vi "Lab Panel V6.00.vi"() -> ()   [LabVIEW 2017]
uses:
  SelectLAB0X-N.ctl
  SIG LAB0X-N.ctl
  Set LAB0X-N.ctl
  <vilib>/Platform/TimedLoop/XDataNode/timing_clust.ctl
  <vilib>/Platform/TimedLoop/XDataNode/nitl_modes.ctl
  <vilib>/Platform/TimedLoop/XDataNode/wakeup.ctl
  Global display 1.vi
  Global display 4.vi
  Global display 3.vi
  Global display 2.vi
  Global 1.vi
  <vilib>/platform/TimedLoop/XDataNode/XDataNode.xnode
  <vilib>/Platform/TimedLoop/XDataNode/XDNodeRunTimeDep.lvlib
panel:
  in  "path to JPEG file":path=path "C:/Users/Mike/Documents/Crabtree/Crabtree/Hardware/crabtree"
  out "Simulate IND":bool
  out "Amb Tp":dbl format="%#.0f"
  out "Tp Up":dbl
  out "network error":bool
  out "TEMP":bool
  out "AI":bool
  in  "stop all":bool
  in  "ADMIN":bool
  in  "Tab Control 2":T1(tab)
  out "SIG LAB05-2":T2 {"PF" format="%.2f"; "AMPS" format="%.1f"}
  out "SIG LAB05-1":T2 {"PF" format="%.2f"; "AMPS" format="%.1f"}
  out "SIG LAB04-2":T2 {"PF" format="%.2f"; "AMPS" format="%.1f"}
  out "SIG LAB04-1":T2 {"PF" format="%.2f"; "AMPS" format="%.1f"}
  out "SIG LAB03-2":T2 {"PF" format="%.2f"; "AMPS" format="%.1f"}
  out "SIG LAB03-1":T2 {"PF" format="%.2f"; "AMPS" format="%.1f"}
  out "SIG LAB02-2":T2 {"PF" format="%.2f"; "AMPS" format="%.1f"}
  in  "RUN LAB01-1":bool
  in  "O/I  LAB05-1":bool
  in  "O/I  LAB05-2":bool
  in  "O/I  LAB04-1":bool
  in  "O/I  LAB04-2":bool
  in  "O/I  LAB02-1":bool
  in  "O/I  LAB02-2":bool
  in  "O/I  LAB01-2":bool
  in  "O/I  LAB01-1":bool
  in  "O/I  LAB03-1":bool
  in  "RUN LAB05-2":bool
  in  "RUN LAB05-1":bool
  in  "RUN LAB04-2":bool
  in  "RUN LAB04-1":bool
  in  "RUN LAB03-2":bool
  in  "RUN LAB03-1":bool
  in  "RUN LAB02-2":bool
  in  "RUN LAB02-1":bool
  in  "RUN LAB01-2":bool
  in  "SELECT LAB05-2":T3
  in  "SELECT LAB05-1":T3
  in  "SELECT LAB04-2":T3
  in  "SELECT LAB04-1":T3
  in  "SELECT LAB03-2":T3
  in  "SELECT LAB03-1":T3
  in  "SELECT LAB02-2":T3
  in  "SELECT LAB02-1":T3
  in  "SELECT LAB01-2":T3
  in  "SELECT LAB01-1":T3
  in  "O/I  LAB03-2":bool
  out "SIG LAB01-1":T2 {"PF" format="%.2f"; "AMPS" format="%.1f"}
  out "SIG LAB01-2":T2 {"PF" format="%.2f"; "AMPS" format="%.1f"}
  out "SIG LAB02-1":T2 {"PF" format="%.2f"; "AMPS" format="%.1f"}
  out "DISP LAB05-2":T4 {"MINS" format="%.2g"}
  out "DISP LAB05-1":T4 {"MINS" format="%.2g"}
  out "DISP LAB04-2":T4 {"MINS" format="%.2g"}
  out "DISP LAB04-1":T4 {"MINS" format="%.2g"}
  out "DISP LAB03-2":T4 {"MINS" format="%.2g"}
  out "DISP LAB03-1":T4 {"MINS" format="%.2g"}
  in  "SET LAB05-2":T5={"NAME"="", "DESCRIPTION"="", "CYCLES"=5.0, "T-RISE mins"=0.0, "T-RISE deg C"=0.0} {"CYCLES" min=5.0 step=1.0}
  in  "SET LAB05-1":T5={"NAME"="", "DESCRIPTION"="", "CYCLES"=5.0, "T-RISE mins"=0.0, "T-RISE deg C"=0.0} {"CYCLES" min=5.0 step=1.0}
  in  "SET LAB04-2":T5={"NAME"="", "DESCRIPTION"="", "CYCLES"=5.0, "T-RISE mins"=0.0, "T-RISE deg C"=0.0} {"CYCLES" min=5.0 step=1.0}
  in  "SET LAB04-1":T5={"NAME"="", "DESCRIPTION"="", "CYCLES"=5.0, "T-RISE mins"=0.0, "T-RISE deg C"=0.0} {"CYCLES" min=5.0 step=1.0}
  in  "SET LAB03-2":T5={"NAME"="", "DESCRIPTION"="", "CYCLES"=5.0, "T-RISE mins"=0.0, "T-RISE deg C"=0.0} {"CYCLES" min=5.0 step=1.0}
  in  "SET LAB03-1":T5={"NAME"="", "DESCRIPTION"="", "CYCLES"=5.0, "T-RISE mins"=0.0, "T-RISE deg C"=0.0} {"CYCLES" min=5.0 step=1.0}
  out "DISP LAB02-2":T4 {"MINS" format="%.2g"}
  out "DISP LAB02-1":T4 {"MINS" format="%.2g"}
  in  "SET LAB02-2":T5={"NAME"="", "DESCRIPTION"="", "CYCLES"=5.0, "T-RISE mins"=0.0, "T-RISE deg C"=0.0} {"CYCLES" min=5.0 step=1.0}
  in  "SET LAB02-1":T5={"NAME"="", "DESCRIPTION"="", "CYCLES"=5.0, "T-RISE mins"=0.0, "T-RISE deg C"=0.0} {"CYCLES" min=5.0 step=1.0}
  out "RESULT LAB05-2":bool
  out "RESULT LAB05-1":bool
  out "RESULT LAB04-2":bool
  out "RESULT LAB04-1":bool
  out "RESULT LAB03-2":bool
  out "RESULT LAB03-1":bool
  out "RESULT LAB02-2":bool
  out "RESULT LAB02-1":bool
  out "RESULT LAB01-2":bool
  out "RESULT LAB01-1":bool
  in  "SET LAB01-1":T6={"NAME"="", "DESCRIPTION"="", "CYCLES"=5.0, "T-RISE mins"=0.0, "T-RISE deg C"=0.0} {"CYCLES" min=5.0 step=1.0}
  in  "SET LAB01-2":T5={"NAME"="", "DESCRIPTION"="", "CYCLES"=5.0, "T-RISE mins"=0.0, "T-RISE deg C"=0.0} {"CYCLES" min=5.0 step=1.0}
  out "DISP LAB01-1":T4 {"MINS" format="%.2g"}
  out "DISP LAB01-2":T4 {"MINS" format="%.2f"}
  out "TEMP RISE LAB05-2":cluster{"TL":dbl, "TN":dbl}
  out "TEMP RISE LAB05-1":cluster{"TL":dbl, "TN":dbl}
  out "TEMP RISE LAB04-2":cluster{"TL":dbl, "TN":dbl}
  out "TEMP RISE LAB04-1":cluster{"TL":dbl, "TN":dbl}
  out "TEMP RISE LAB03-2":cluster{"TL":dbl, "TN":dbl}
  out "TEMP RISE LAB03-1":cluster{"TL":dbl, "TN":dbl}
  out "TEMP RISE LAB02-2":cluster{"TL":dbl, "TN":dbl}
  out "TEMP RISE LAB02-1":cluster{"TL":dbl, "TN":dbl}
  out "TEMP RISE LAB01-2":cluster{"TL":dbl, "TN":dbl}
  out "TEMP RISE LAB01-1":cluster{"TL":dbl, "TN":dbl}
  out "JIG LAB05-2":bool
  out "JIG LAB05-1":bool
  out "JIG LAB04-2":bool
  out "JIG LAB04-1":bool
  out "JIG LAB03-2":bool
  out "JIG LAB03-1":bool
  out "JIG LAB02-2":bool
  out "JIG LAB02-1":bool
  out "JIG LAB01-2":bool
  out "JIG LAB01-1":bool
  out "TEMP START LAB01-1":cluster{"TL":dbl, "TN":dbl}
  out "TEMP START LAB02-1":cluster{"TL":dbl, "TN":dbl}
  out "TEMP START LAB03-1":cluster{"TL":dbl, "TN":dbl}
  out "TEMP START LAB04-1":cluster{"TL":dbl, "TN":dbl}
  out "TEMP START LAB01-2":cluster{"TL":dbl, "TN":dbl}
  out "TEMP START LAB02-2":cluster{"TL":dbl, "TN":dbl}
  out "TEMP START LAB03-2":cluster{"TL":dbl, "TN":dbl}
  out "TEMP START LAB04-2":cluster{"TL":dbl, "TN":dbl}
  out "TEMP START LAB05-2":cluster{"TL":dbl, "TN":dbl}
  out "TEMP START LAB05-1":cluster{"TL":dbl, "TN":dbl}
  out "LOG LAB05-2":string
  out "LOG LAB04-2":string
  out "LOG LAB03-2":string
  out "LOG LAB02-2":string
  out "LOG LAB01-2":string
  out "LOG LAB05-1":string
  out "LOG LAB04-1":string
  out "LOG LAB03-1":string
  out "LOG LAB02-1":string
  out "LOG LAB01-1":string
  in  "Tab charts":T7(tab)
  out "LAB01 VOLTS":dynamicdata(graph)
  out "LAB01 AMPS":dynamicdata(graph)
  out "LAB01 deg C":dynamicdata(graph)
  out "LAB02 VOLTS":dynamicdata(graph)
  out "LAB02 AMPS":dynamicdata(graph)
  out "LAB02 deg C":dynamicdata(graph)
  out "LAB03 VOLTS":dynamicdata(graph)
  out "LAB03 AMPS":dynamicdata(graph)
  out "LAB03 deg C":dynamicdata(graph)
  out "LAB04 VOLTS":dynamicdata(graph)
  out "LAB04 AMPS":dynamicdata(graph)
  out "LAB04 deg C":dynamicdata(graph)
  out "LAB05 VOLTS":dynamicdata(graph)
  out "LAB05 AMPS":dynamicdata(graph)
  out "LAB05 deg C":dynamicdata(graph)
  out "Reset Error":bool
  out "Er USB#2":dbl
  out "Er USB#1":dbl
  out "Er USB#0":dbl
  out "Resets Done":dbl
  out "Error USB #2":bool
  out "Error USB #1":bool
  out "Error USB #0":bool
  in  "MAIL SETTINGS":T8
  out "MAIL REPORT":string
  in  "TO (string):":string
  in  "Send Mail Now":bool
  in  "Auto Mail Send":bool
  in  "Network Directory":path
  in  "JIG ON TIME (S)":dbl=1.0 min=1.0 max=10.0 step=0.5 format="%.1g"
  in  "JIG OFF TIME (S)":dbl=2.0 min=2.0 max=10.0 step=0.5 format="%.1g"
  in  "Reset Measuring":bool
  out "path":path
  out "JIG RELAY CYCLES":T9
  out "ON L05-2":cluster{"amps":dbl, "volts":dbl, "pf":dbl}
  out "ON L05-1":cluster{"amps":dbl, "volts":dbl, "pf":dbl}
  out "FAIL LAB05-2":cluster{"LO":dbl, "HI":dbl}
  out "FAIL LAB05-1":cluster{"LO":dbl, "HI":dbl}
  out "FAIL LAB04-2":cluster{"LO":dbl, "HI":dbl}
  out "FAIL LAB04-1":cluster{"LO":dbl, "HI":dbl}
  out "FAIL LAB03-2":cluster{"LO":dbl, "HI":dbl}
  out "FAIL LAB03-1":cluster{"LO":dbl, "HI":dbl}
  out "FAIL LAB02-2":cluster{"LO":dbl, "HI":dbl}
  out "FAIL LAB02-1":cluster{"LO":dbl, "HI":dbl}
  out "FAIL LAB01-2":cluster{"LO":dbl, "HI":dbl}
  out "FAIL LAB01-1":cluster{"LO":dbl, "HI":dbl}
  out "ON L01-1":cluster{"amps":dbl, "volts":dbl, "pf":dbl}
  out "ON L01-2":cluster{"amps":dbl, "volts":dbl, "pf":dbl}
  out "ON L02-1":cluster{"amps":dbl, "volts":dbl, "pf":dbl}
  out "ON L02-2":cluster{"amps":dbl, "volts":dbl, "pf":dbl}
  out "ON L03-1":cluster{"amps":dbl, "volts":dbl, "pf":dbl}
  out "ON L03-2":cluster{"amps":dbl, "volts":dbl, "pf":dbl}
  out "ON L04-1":cluster{"amps":dbl, "volts":dbl, "pf":dbl}
  out "ON L04-2":cluster{"amps":dbl, "volts":dbl, "pf":dbl}
  in  "Open Com Port":bool
  out "LA05-2 (TN)":bool
  out "LA05-2 (TL)":bool
  out "LA05-1 (TN)":bool
  out "LA05-1 (TL)":bool
  out "LA04-2 (TN)":bool
  out "LA04-2 (TL)":bool
  out "LA04-1 (TN)":bool
  out "LA04-1 (TL)":bool
  out "LA03-2 (TN)":bool
  out "LA03-2 (TL)":bool
  out "LA03-1 (TN)":bool
  out "LA03-1 (TL)":bool
  out "LA02-2 (TN)":bool
  out "LA02-2 (TL)":bool
  out "LA02-1 (TN)":bool
  out "LA02-1 (TL)":bool
  out "LA01-2 (TN)":bool
  out "LA01-2 (TL)":bool
  out "LA01-1 (TN)":bool
  out "LA01-1 (TL)":bool
  out "TEMP LA05":T10
  out "TEMP LA04":T10
  out "TEMP LA03":T10
  out "TEMP LA02":T10
  out "TEMP LA01":T10
  out "Ref deg C":dbl format="%#.0f"
  out "Temp read loop":dbl
  out "Com Port Status":bool
  out "Com setup loops":i32
  out "VISA Com out":refnum<visa-resource-name>
  in  "Select COM port":refnum<visa-resource-name>="COM6"
  in  "Read Temp":bool
  out "Error Temp":bool
  out "AI Task":bool
  out "AI Task2":dbl
  out "AI Task1":dbl
  out "AI Task0":dbl
  out "Total USB resets":dbl
  in  "Auto Reset":bool
  in  "Mail Test File To:":string
  in  "Mail Test Fail":bool
  out "graph flag":bool
  in  "Temp Test Cal":dbl
  in  "Amps Fail level":dbl
  in  "Fail Loops":dbl
  out "Save JC":bool
  in  "Simulate":bool
  in  "Temp Value":dbl
  in  "Temp Delay Lps":dbl
  in  "SAMPLES":dbl
  in  "RATE (Hz)":dbl
  in  "JIG TEST":T11
  in  "C drive data root dir":path
  out "run lab05-2":bool
  out "run lab05-1":bool
  out "run lab04-2":bool
  out "run lab04-1":bool
  out "run lab03-2":bool
  out "run lab03-1":bool
  out "run lab02-2":bool
  out "run lab02-1":bool
  out "run lab01-2":bool
  out "run lab01-1":bool
  in  "Tab Control":T12(tab)
  out "LAB01-2 (GRAPH)":dynamicdata(graph)
  out "LAB01-1 (GRAPH)":dynamicdata(graph)
  out "LAB02-2 (GRAPH)":dynamicdata(graph)
  out "LAB02-1 (GRAPH)":dynamicdata(graph)
  out "LAB03-2 (GRAPH)":dynamicdata(graph)
  out "LAB03-1 (GRAPH)":dynamicdata(graph)
  out "LAB04-2 (GRAPH)":dynamicdata(graph)
  out "LAB04-1 (GRAPH)":dynamicdata(graph)
  out "LAB05-2 (GRAPH)":dynamicdata(graph)
  out "LAB05-1 (GRAPH)":dynamicdata(graph)
  out "Any Test Running":bool
  out "Read Time":dbl
  out "LAB05 TEMP":T13
  out "LAB04 TEMP":T13
  out "LAB02 TEMP":T13
  out "LAB01 TEMP":T13
  out "LAB03 TEMP":T13
  out "LAB05-TP":bool
  out "LAB04-TP":bool
  out "LAB03-TP":bool
  out "LAB02-TP":bool
  out "LAB01-TP":bool
  out "Analog error":bool
  out "USB OUT 0":bool[](array[boolean])
  out "USB OUT 1":bool[](array[boolean])
  out "USB OUT 2":bool[](array[boolean])
  in  "Ambient Volts":dbl format="%.2f"
  in  "PF":dbl min=0.0 max=1.0 step=0.1 format="%#.1f"
  in  "VOLTS":dbl
  in  "OFF amps":dbl min=0.0 max=100.0 step=0.1 format="%#.1f"
  in  "ON amps":dbl
  in  "LAB deg C":T14
  out "AI data 0":waveform(dbl)[](array[waveform])
  out "AI data 1":waveform(dbl)[](array[waveform])
  out "AI data 2":waveform(dbl)[](array[waveform])
  out "AI Error":errorcluster[](array[cluster])
  out "AI loop time":dbl format="%.6g"
  out "loops":dbl
  out "on loops":dbl format="%#.0f"
  out "off loops":dbl format="%#.0f"
  out "jig cycle":dbl
  out "TDMS LAB01-1":refnum<k34>
  out "data file error":errorcluster
  out "TDMS LAB02-1":refnum<k34>
  out "TDMS LAB01-2":refnum<k34>
  out "TDMS LAB02-2":refnum<k34>
  out "TDMS LAB03-1":refnum<k34>
  out "TDMS LAB03-2":refnum<k34>
  out "TDMS LAB04-1":refnum<k34>
  out "TDMS LAB04-2":refnum<k34>
  out "TDMS LAB05-1":refnum<k34>
  out "TDMS LAB05-2":refnum<k34>
  out "mail control":string
  out "File Time Stamp":timestamp
  in  "stop":bool
  out "deg C (volts)":dbl
  out "Application Directory":path
  out "TEMP REF cal":dbl
  out "CAL LAB01":T15 {"2 (TN) cal" min=0.0 step=0.01 format="%.2f"; "2 (TL) cal" min=0.0 step=0.01 format="%.2f"; "2 (PF) cal" min=0.0 step=0.01 format="%.2f"; "2 (V) cal" min=0.0 step=0.01 format="%.2f"; "2 (A) cal" min=0.0 step=0.01 format="%.2f"; "1 (TN) cal" min=0.0 step=0.01 format="%.2f"; "1 (TL) cal" min=0.0 step=0.01 format="%.2f"; "1 (PF) cal" min=0.0 step=0.01 format="%.2f"; "1 (V) cal" min=0.0 step=0.01 format="%.2f"; "1  (A) cal" min=0.0 step=0.01 format="%.2f"}
  out "CAL LAB03":T15 {"2 (TN) cal" min=0.0 step=0.01 format="%.2f"; "2 (TL) cal" min=0.0 step=0.01 format="%.2f"; "2 (PF) cal" min=0.0 step=0.01 format="%.2f"; "2 (V) cal" min=0.0 step=0.01 format="%.2f"; "2 (A) cal" min=0.0 step=0.01 format="%.2f"; "1 (TN) cal" min=0.0 step=0.01 format="%.2f"; "1 (TL) cal" min=0.0 step=0.01 format="%.2f"; "1 (PF) cal" min=0.0 step=0.01 format="%.2f"; "1 (V) cal" min=0.0 step=0.01 format="%.2f"; "1  (A) cal" min=0.0 step=0.01 format="%.2f"}
  out "CAL LAB02":T16 {"2 (TN) cal" min=0.0 step=0.01 format="%.2f"; "2 (TL) cal" min=0.0 step=0.01 format="%.2f"; "2 (PF) cal" min=0.0 step=0.01 format="%.2f"; "2 (V) cal" min=0.0 step=0.01 format="%.2f"; "2 (A) cal" min=0.0 step=0.01 format="%.2f"; "1 (TN) cal" min=0.0 step=0.01 format="%.2f"; "1 (TL) cal" min=0.0 step=0.01 format="%.2f"; "1 (PF) cal" min=0.0 step=0.01 format="%.2f"; "1 (V) cal" min=0.0 step=0.01 format="%.2f"; "1 (A) cal" min=0.0 step=0.01 format="%.2f"}
  out "CAL LAB05":T15 {"2 (TN) cal" min=0.0 step=0.01 format="%.2f"; "2 (TL) cal" min=0.0 step=0.01 format="%.2f"; "2 (PF) cal" min=0.0 step=0.01 format="%.2f"; "2 (V) cal" min=0.0 step=0.01 format="%.2f"; "2 (A) cal" min=0.0 step=0.01 format="%.2f"; "1 (TN) cal" min=0.0 step=0.01 format="%.2f"; "1 (TL) cal" min=0.0 step=0.01 format="%.2f"; "1 (PF) cal" min=0.0 step=0.01 format="%.2f"; "1 (V) cal" min=0.0 step=0.01 format="%.2f"; "1  (A) cal" min=0.0 step=0.01 format="%.2f"}
  out "CAL LAB04":T15 {"2 (TN) cal" min=0.0 step=0.01 format="%.2f"; "2 (TL) cal" min=0.0 step=0.01 format="%.2f"; "2 (PF) cal" min=0.0 step=0.01 format="%.2f"; "2 (V) cal" min=0.0 step=0.01 format="%.2f"; "2 (A) cal" min=0.0 step=0.01 format="%.2f"; "1 (TN) cal" min=0.0 step=0.01 format="%.2f"; "1 (TL) cal" min=0.0 step=0.01 format="%.2f"; "1 (PF) cal" min=0.0 step=0.01 format="%.2f"; "1 (V) cal" min=0.0 step=0.01 format="%.2f"; "1  (A) cal" min=0.0 step=0.01 format="%.2f"}
  out "cal file error out":errorcluster
  in  "SET (cal)":bool
  out "AI Data 0":waveform(dbl)[](graph)
  out "AI Data 1":waveform(dbl)[](graph)
  out "AI Data 2":waveform(dbl)[](graph)
  # "http://Mike:8000/Lab%20Panel%20V6.0.html"
  # "LAB01"
  # "LAB02"
  # "LAB03"
  # "LAB04"
  # "LAB05"
  # "LAB01"
  # "LAB02"
  # "LAB03"
  # "LAB04"
  # "LAB05"
  # "PANEL ID / DATE / TIME / NAME / DESCRIPTION / CYCLES / TEST TIME / STATUS"
  # "PANEL ID / DATE / TIME / NAME / DESCRIPTION / CYCLES / TEST TIME / STATUS"
  # "http://This IP:8000/Lab_Panel"
  # "(Enter recipients address seperated by comma)"
  # "JIG SET"
  # "Temperature circuits \ndetected at start up."
  # "PANEL CONTROL TO BE ON"
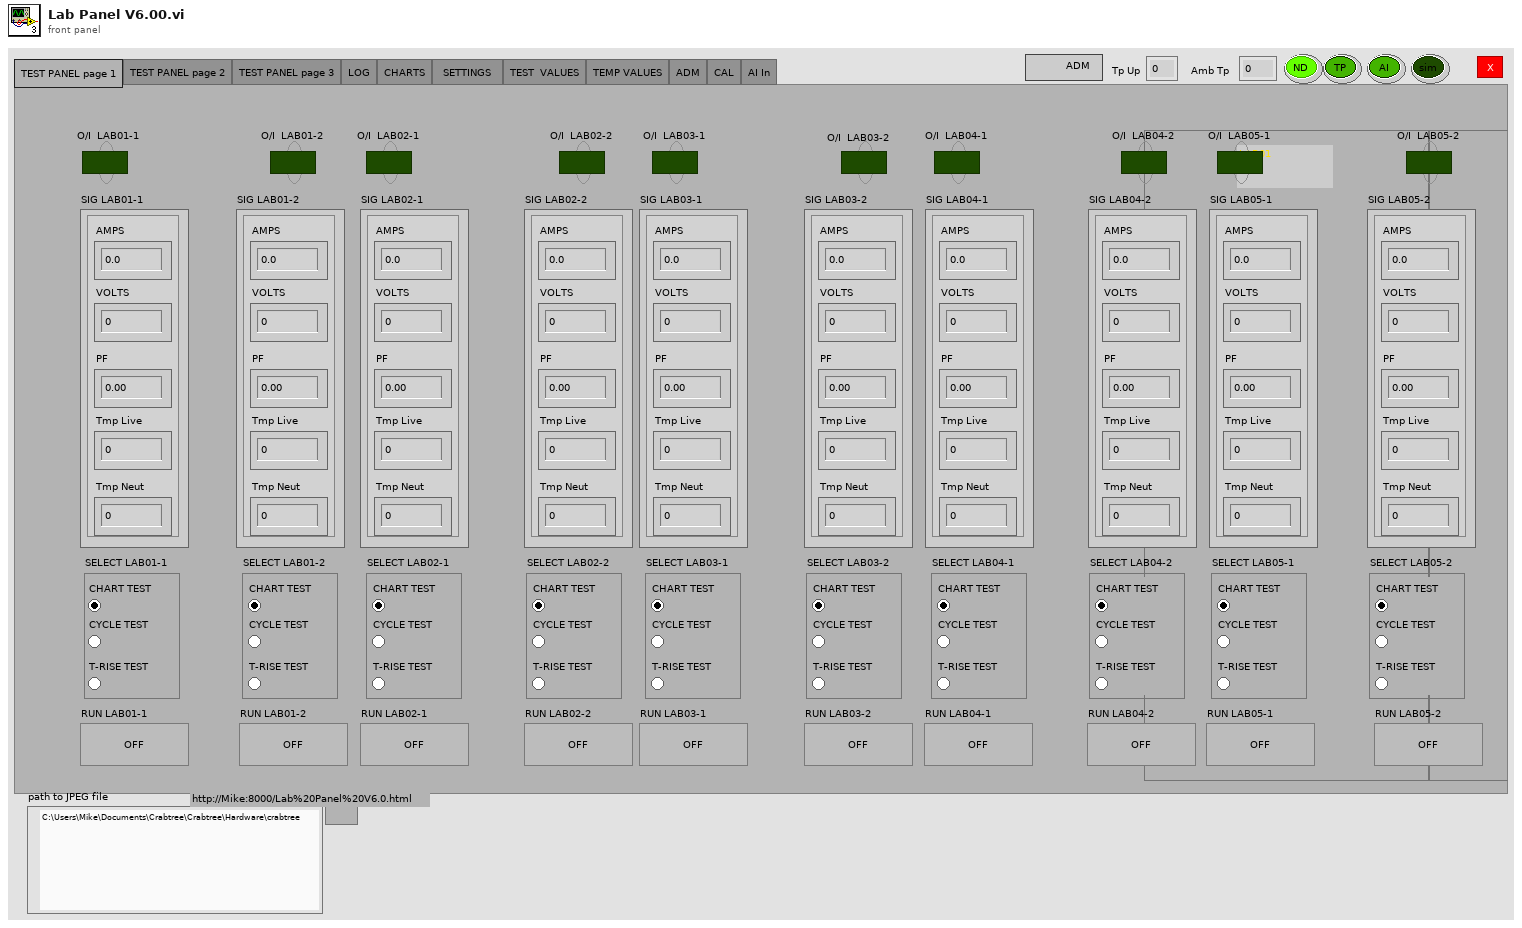
[diagram p1: front panel]
types:
  T1 = enum32{"TEST PANEL page 1", "TEST PANEL page 2", "TEST PANEL page 3", "LOG", "CHARTS", "SETTINGS   ", "TEST  VALUES", "TEMP VALUES", "ADM", "CAL", "AI In"}
  T2 = typedef "SIG LAB0X-N.ctl" = cluster{"AMPS":dbl, "VOLTS":dbl, "PF":dbl, "Tmp Live":dbl, "Tmp Neut":dbl}
  T3 = typedef "SelectLAB0X-N.ctl" = enum32{"CHART TEST", "CYCLE TEST", "T-RISE TEST"}
  T4 = cluster{"CYCLE":dbl, "MINS":dbl, "STATUS":string}
  T5 = cluster{"NAME":string, "DESCRIPTION":string, "CYCLES":dbl, "T-RISE mins":dbl, "T-RISE deg C":dbl}
  T6 = typedef "Set LAB0X-N.ctl" = cluster{"NAME":string, "DESCRIPTION":string, "CYCLES":dbl, "T-RISE mins":dbl, "T-RISE deg C":dbl}
  T7 = enum32{"LAB01", "LAB02", "LAB03", "LAB04", "LAB05"}
  T8 = cluster{"OUT SERVER ADDRESS":string, "FROM ACCOUNT":string, "USER NAME":string, "PASSWORD":string, "TEST MAIL":bool, "TEST MAIL STATUS":string, "mail error":errorcluster}
  T9 = cluster{"LAB01-1":dbl, "LAB01-2":dbl, "LAB02-1":dbl, "LAB02-2":dbl, "LAB03-1":dbl, "LAB03-2":dbl, "LAB04-1":dbl, "LAB04-2":dbl, "LAB05-1":dbl, "LAB05-2":dbl}
  T10 = cluster{"TL-1":dbl, "TN-1":dbl, "TL-2":dbl, "TN-2":dbl, "TL -1COUNT":dbl, "TN-1 COUNT":dbl, "TL-2 COUNT":dbl, "TN-2 COUNT":dbl}
  T11 = cluster{" LAB01-1":bool, " LAB01-2":bool, "LAB02-1":bool, " LAB02-2":bool, "LAB03-1":bool, "LAB03-2":bool, "LAB04-1":bool, "LAB04-2":bool, "LAB05-1":bool, "LAB05-2":bool}
  T12 = enum32{"LAB01", "LAB02", "LAB03", "LAB04", "LAB05", "TEMPERATURE", "GENERAL INFO", "Simulate", "AI Data Out"}
  T13 = cluster{"T1 Live":dbl, "T1 Neut":dbl, "T2 Live":dbl, "T2 Neut":dbl, "ID":dbl, "ER":dbl}
  T14 = cluster{"1 TL":dbl, "1 TN":dbl, "2 TL":dbl, "2 TN":dbl, "ID":dbl, "ER":dbl}
  T15 = cluster{"1  (A) cal":dbl, "1 (V) cal":dbl, "1 (PF) cal":dbl, "1 (TL) cal":dbl, "1 (TN) cal":dbl, "2 (A) cal":dbl, "2 (V) cal":dbl, "2 (PF) cal":dbl, "2 (TL) cal":dbl, "2 (TN) cal":dbl}
  T16 = cluster{"1 (A) cal":dbl, "1 (V) cal":dbl, "1 (PF) cal":dbl, "1 (TL) cal":dbl, "1 (TN) cal":dbl, "2 (A) cal":dbl, "2 (V) cal":dbl, "2 (PF) cal":dbl, "2 (TL) cal":dbl, "2 (TN) cal":dbl}
  T17 = enum8{"Enabled", "Disabled", "Disabled and Grayed Out"}
  T18 = enum16{"open", "replace", "create", "open or create", "replace or create", "replace or create with confirmation"}
  T19 = typedef "XDNodeRunTimeDep.lvlib/timing_clust.ctl" = cluster{"Expected End [f-1]":u64, "Actual End [f-1]":u64, "Finished Late? [f-1]":bool, "Expected End [i-1]":u64, "Actual End [i-1]":u64, "Finished Late? [i-1]":bool, "Expected Start [i]":u64, "Actual Start [i]":u64, "Expected Start [f]":u64, "Actual Start [f]":u64, "Source Name":string, "Structure Name":string, "Period":i64, "Deadline":i64, "Offset":i64, "Start":i64, "Priority":i32, "Timeout":i32, "Mode":T20, "Wakeup Reason":T21, "Error":errorcluster, "Source Type":string, "Secondary Source Type":string, "Global End Time":u64, "Global Start Time":u64, "Frame Duration":u64, "Iteration Duration":u64, "Assigned CPU":i32, "I/O Scan Engine Mode":u32}
  T20 = typedef "XDNodeRunTimeDep.lvlib/nitl_modes.ctl" = enum32{"No Change", "Process missed periods, maintain original phase", "Discard missed periods, maintain original phase", "Process missed periods, ignore original phase", "Discard missed periods, ignore original phase"}
  T21 = typedef "XDNodeRunTimeDep.lvlib/wakeup.ctl" = enum32{"Normal", "Aborted", "Asynchronous wakeup", "Timing source error", "Timed loop error", "Timeout"}
  T22 = enum16{"open", "open or create", "create or replace", "create", "open (read-only)"}
  T23 = cluster{"status":string, "mail server":string, "mail from":string, "mail to":string, "mail file":bool}
  T24 = cluster{"SET LAB01-1":T6, "SET LAB01-2":cluster{"NAME":string, "DESCRIPTION":string, "CYCLES":dbl, "T-RISE mins":dbl, "T-RISE deg C":dbl}, "SET LAB02-1":cluster{"NAME":string, "DESCRIPTION":string, "CYCLES":dbl, "T-RISE mins":dbl, "T-RISE deg C":dbl}, "SET LAB02-2":cluster{"NAME":string, "DESCRIPTION":string, "CYCLES":dbl, "T-RISE mins":dbl, "T-RISE deg C":dbl}, "SET LAB03-1":cluster{"NAME":string, "DESCRIPTION":string, "CYCLES":dbl, "T-RISE mins":dbl, "T-RISE deg C":dbl}, "SET LAB03-2":cluster{"NAME":string, "DESCRIPTION":string, "CYCLES":dbl, "T-RISE mins":dbl, "T-RISE deg C":dbl}, "SET LAB04-1":cluster{"NAME":string, "DESCRIPTION":string, "CYCLES":dbl, "T-RISE mins":dbl, "T-RISE deg C":dbl}, "SET LAB04-2":cluster{"NAME":string, "DESCRIPTION":string, "CYCLES":dbl, "T-RISE mins":dbl, "T-RISE deg C":dbl}, "SET LAB05-1":cluster{"NAME":string, "DESCRIPTION":string, "CYCLES":dbl, "T-RISE mins":dbl, "T-RISE deg C":dbl}, "SET LAB05-2":cluster{"NAME":string, "DESCRIPTION":string, "CYCLES":dbl, "T-RISE mins":dbl, "T-RISE deg C":dbl}, "Network Directory":path, "C drive data root dir":path, "RATE (Hz)":dbl, "SAMPLES":dbl, "Select COM port":refnum<visa-resource-name>, "Temp Delay Lps":dbl, "Temp Value":dbl, "Fail Loops":dbl, "Temp Test Cal":dbl, "Amps Fail level":dbl, "Mail Test File To:":string, "Mail Test Fail":bool}
  T25 = cluster{"MAIL SETTINGS":cluster{"OUT SERVER ADDRESS":string, "FROM ACCOUNT":string, "USER NAME":string, "PASSWORD":string, "TEST MAIL":bool, "TEST MAIL STATUS":string, "mail error":errorcluster}, "Auto Mail Send":bool, string}
  T26 = cluster{"id1":bool, "id2":bool, "id3":bool, "id4":bool, "id5":bool}
  T27 = cluster{"T1":dbl, "T2":dbl, "T3":dbl, "T4":dbl, "ID":dbl, "ER":dbl}
  T28 = typedef "imagedata.ctl" = cluster{"image type":i32, "image depth":i32, "image":u8[], "mask":u8[], "colors":u32[], "Rectangle":cluster{"left":i16, "top":i16, "right":i16, "bottom":i16}}
  T29 = cluster{"STATUS":string, "OUT SERVER ADDRESS":string, "FROM ACCOUNT":string, "Mail Test File To:":string, "Mail Test Fail":bool}
  T30 = cluster{"LAB01-1 (A)":dbl, "LAB01-1 (V)":dbl, "LAB01-1 (PF)":dbl, "LAB01-2 (A)":dbl, "LAB01-2 (V)":dbl, "LAB01-2 (PF)":dbl}
  T31 = cluster{"LAB02-1 (A)":dbl, "LAB02-1 (V)":dbl, "LAB02-1 (PF)":dbl, "LAB02-2 (A)":dbl, "LAB02-2 (V)":dbl, "LAB02-2 (PF)":dbl}
  T32 = cluster{"LAB03-1 (A)":dbl, "LAB03-1 (V)":dbl, "LAB03-1 (PF)":dbl, "LAB03-2 (A)":dbl, "LAB03-2 (V)":dbl, "LAB03-2 (PF)":dbl}
  T33 = cluster{"LAB04-1 (A)":dbl, "LAB04-1 (V)":dbl, "LAB04-1 (PF)":dbl, "LAB04-2 (A)":dbl, "LAB04-2 (V)":dbl, "LAB04-2 (PF)":dbl}
  T34 = cluster{"LAB05-1 (A)":dbl, "LAB05-1 (V)":dbl, "LAB05-1 (PF)":dbl, "LAB05-2 (A)":dbl, "LAB05-2 (V)":dbl, "LAB05-2 (PF)":dbl}
  T35 = cluster{"OFF amps":dbl, "VOLTS":dbl, "PF":dbl, "OFF amps":dbl, "VOLTS":dbl, "PF":dbl}
  T36 = cluster{"FAIL LAB01-1":cluster{"LO":dbl, "HI":dbl}, "SIG LAB01-1":T2, "TEMP START LAB01-1":cluster{"TL":dbl, "TN":dbl}, "DISP LAB01-1":cluster{"CYCLE":dbl, "MINS":dbl, "STATUS":string}, "SET LAB01-1":T6, "TDMS LAB01-1":refnum<k34>}
  T37 = cluster{"FAIL LAB01-2":cluster{"LO":dbl, "HI":dbl}, "SIG LAB01-2":T2, "TEMP START LAB01-2":cluster{"TL":dbl, "TN":dbl}, "DISP LAB01-2":cluster{"CYCLE":dbl, "MINS":dbl, "STATUS":string}, "SET LAB01-2":cluster{"NAME":string, "DESCRIPTION":string, "CYCLES":dbl, "T-RISE mins":dbl, "T-RISE deg C":dbl}, "TDMS LAB01-2":refnum<k34>}
  T38 = cluster{"FAIL LAB02-1":cluster{"LO":dbl, "HI":dbl}, "SIG LAB02-1":T2, "TEMP START LAB02-1":cluster{"TL":dbl, "TN":dbl}, "DISP LAB02-1":cluster{"CYCLE":dbl, "MINS":dbl, "STATUS":string}, "SET LAB02-1":cluster{"NAME":string, "DESCRIPTION":string, "CYCLES":dbl, "T-RISE mins":dbl, "T-RISE deg C":dbl}, "TDMS LAB02-1":refnum<k34>}
  T39 = cluster{"FAIL LAB02-2":cluster{"LO":dbl, "HI":dbl}, "SIG LAB02-2":T2, "TEMP START LAB02-2":cluster{"TL":dbl, "TN":dbl}, "DISP LAB02-2":cluster{"CYCLE":dbl, "MINS":dbl, "STATUS":string}, "SET LAB02-2":cluster{"NAME":string, "DESCRIPTION":string, "CYCLES":dbl, "T-RISE mins":dbl, "T-RISE deg C":dbl}, "TDMS LAB02-2":refnum<k34>}
  T40 = cluster{"FAIL LAB03-1":cluster{"LO":dbl, "HI":dbl}, "SIG LAB03-1":T2, "TEMP START LAB03-1":cluster{"TL":dbl, "TN":dbl}, "DISP LAB03-1":cluster{"CYCLE":dbl, "MINS":dbl, "STATUS":string}, "SET LAB03-1":cluster{"NAME":string, "DESCRIPTION":string, "CYCLES":dbl, "T-RISE mins":dbl, "T-RISE deg C":dbl}, "TDMS LAB03-1":refnum<k34>}
  T41 = cluster{"FAIL LAB03-2":cluster{"LO":dbl, "HI":dbl}, "SIG LAB03-2":T2, "TEMP START LAB03-2":cluster{"TL":dbl, "TN":dbl}, "DISP LAB03-2":cluster{"CYCLE":dbl, "MINS":dbl, "STATUS":string}, "SET LAB03-2":cluster{"NAME":string, "DESCRIPTION":string, "CYCLES":dbl, "T-RISE mins":dbl, "T-RISE deg C":dbl}, "TDMS LAB03-2":refnum<k34>}
  T42 = cluster{"FAIL LAB04-1":cluster{"LO":dbl, "HI":dbl}, "SIG LAB04-1":T2, "TEMP START LAB04-1":cluster{"TL":dbl, "TN":dbl}, "DISP LAB04-1":cluster{"CYCLE":dbl, "MINS":dbl, "STATUS":string}, "SET LAB04-1":cluster{"NAME":string, "DESCRIPTION":string, "CYCLES":dbl, "T-RISE mins":dbl, "T-RISE deg C":dbl}, "TDMS LAB04-1":refnum<k34>}
  T43 = cluster{"FAIL LAB04-2":cluster{"LO":dbl, "HI":dbl}, "SIG LAB04-2":T2, "TEMP START LAB04-2":cluster{"TL":dbl, "TN":dbl}, "DISP LAB04-2":cluster{"CYCLE":dbl, "MINS":dbl, "STATUS":string}, "SET LAB04-2":cluster{"NAME":string, "DESCRIPTION":string, "CYCLES":dbl, "T-RISE mins":dbl, "T-RISE deg C":dbl}, "TDMS LAB04-2":refnum<k34>}
  T44 = cluster{"FAIL LAB05-1":cluster{"LO":dbl, "HI":dbl}, "SIG LAB05-1":T2, "TEMP START LAB05-1":cluster{"TL":dbl, "TN":dbl}, "DISP LAB05-1":cluster{"CYCLE":dbl, "MINS":dbl, "STATUS":string}, "SET LAB05-1":cluster{"NAME":string, "DESCRIPTION":string, "CYCLES":dbl, "T-RISE mins":dbl, "T-RISE deg C":dbl}, "TDMS LAB05-1":refnum<k34>}
  T45 = cluster{"FAIL LAB05-2":cluster{"LO":dbl, "HI":dbl}, "SIG LAB05-2":T2, "TEMP START LAB05-2":cluster{"TL":dbl, "TN":dbl}, "DISP LAB05-2":cluster{"CYCLE":dbl, "MINS":dbl, "STATUS":string}, "SET LAB05-2":cluster{"NAME":string, "DESCRIPTION":string, "CYCLES":dbl, "T-RISE mins":dbl, "T-RISE deg C":dbl}, "TDMS LAB05-2":refnum<k34>}
  T46 = cluster{"MAIL SETTINGS":cluster{"OUT SERVER ADDRESS":string, "FROM ACCOUNT":string, "USER NAME":string, "PASSWORD":string, "TEST MAIL":bool, "TEST MAIL STATUS":string, "mail error":errorcluster}, "Auto Mail Send":bool, "TO (string):":string}
  T47 = cluster{"TP1-L":dbl, "TP1-N":dbl, "TP2-L":dbl, "TP2-N":dbl, "TP1-L COUNT":dbl, "TP1-N COUNT":dbl, "TP2-L COUNT":dbl, "TP2-N COUNT":dbl}
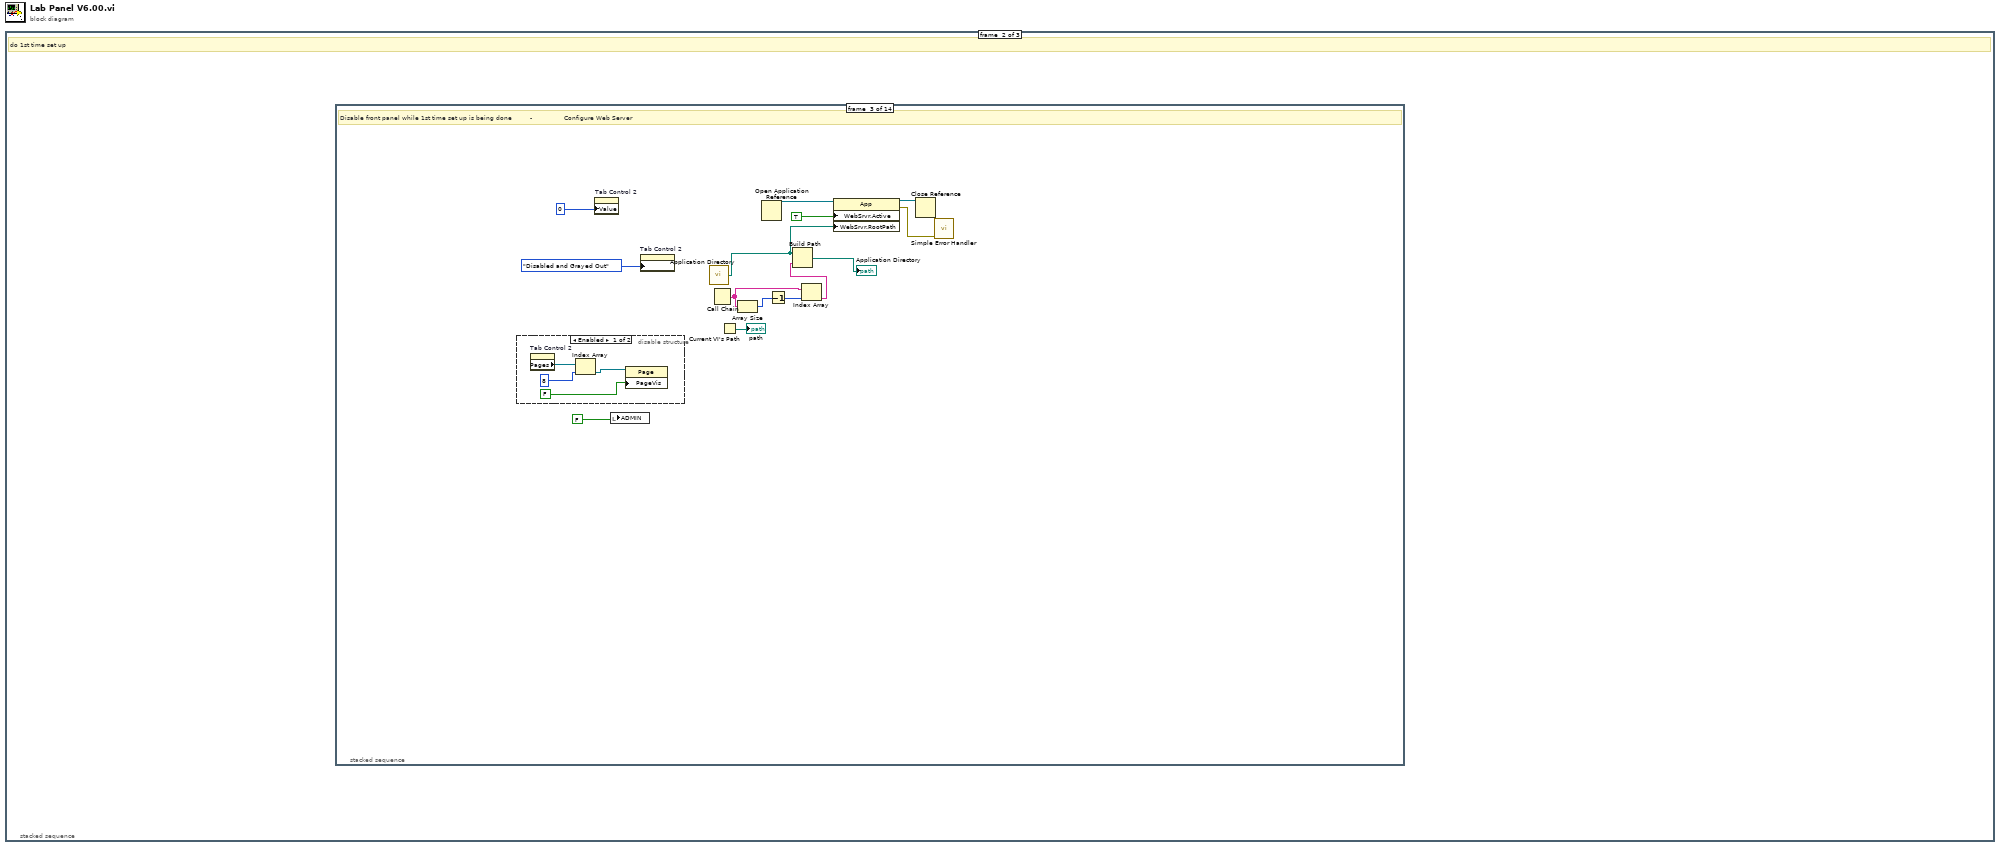
[diagram p0: block diagram]
diagram:
  n1 = stacked-sequence {
    frame #0 {
      # "Front panel Terminals (???)"
      n2 = local write "Save JC"(FALSE) -> ()
      "jig cycle" <- 0
    }
    frame #1 {
      # "do 1st time set up"
      n3 = stacked-sequence {
        frame #0 {
          # "check for simulate mode"
          n4 = call "subvi-simulate v1.vi"() -> ("Sim"=w3:bool)  [unwired: 11 in]
          n5 = case shown="True" w3 {
            frame False {
            }
            frame True {
              n6 = local write "Simulate"(TRUE) -> ()
            }
          }
        }
        frame #1 {
          # "RESET USB AND TEMPERATURE CIRCUITS"
          n7 = local read "Simulate"() -> (w5:bool)
          n8 = case shown="False" w5 {
            frame False {
              n9 = call "Reset USB&temp v 1.vi"() -> ()  [unwired: 11 in, 1 out]
            }
            frame True {
            }
          }
        }
        frame #2 {
          # "Disable front panel while 1st time set up is being done         -                Configure Web Server"
          n10 = disable-structure shown="Enabled" {
            frame Enabled {
              n11 = property on="Tab Control 2" class="TabCtl (strict)"() -> ("Pages"=w23:refnum<vi>[])  [unwired: 2 in, 2 out]
              n12 = Index Array(array=w23, index=8) -> (element=w21:refnum<vi>)
              n13 = property class="Page"(reference=w21, "PageVis"=FALSE) -> ()  [unwired: 1 in, 2 out]
            }
            frame Disabled {
            }
          }
          n14 = property on="Tab Control 2" class="TabCtl (strict)"("Value"=0) -> ()  [unwired: 2 in, 2 out]
          n15 = local write "ADMIN"(FALSE) -> ()
          n16 = property on="Tab Control 2" class="TabCtl (strict)"("DisabledEnum"=T17."Disabled and Grayed Out" ("Disabled")) -> ()  [unwired: 2 in, 2 out]
          n17 = call <vilib>:"Application Directory.vi"() -> ("Application Directory"=w6:path)
          n18 = Call Chain() -> (call chain=w9:string[])
          n19 = Current VI's Path() -> (path=→"path":path)
          n20 = Array Size(array=w9) -> (size(s)=w11:i32)
          n21 = Open Application Reference() -> (3:w16:refnum<vi>)  [unwired: 4 in, 1 out]
          n22 = Decrement(x=w11) -> (x-1=w10:i32)
          n23 = Index Array(array=w9, index=w10) -> (element=w8:string)
          n24 = Build Path(base path=w6, name or relative path=w8) -> (appended path=→"Application Directory":path)
          n25 = property class="App"(reference=w16, "WebSrvr.Active"=TRUE ("Web Server:Server Active"), "WebSrvr.RootPath"=w6) -> (reference out=w14:refnum<vi>, error out=w12:errorcluster)  [unwired: 1 in]
          n26 = Close Reference(reference=w14) -> ()  [unwired: 1 in, 1 out]
          n27 = call <vilib>:"Simple Error Handler.vi"("error in (no error)"=w12) -> ()  [unwired: 4 in, 5 out]
        }
        frame #3 {
          # "Get calibration values"
          n28 = call "sub vi - get calibration values v1.vi"() -> ("TEMP REF CAL"=w24:dbl, "LAB01 (CAL)"=→"CAL LAB01":T15, "LAB02 (CAL)"=→"CAL LAB02":T16, "LAB03 (CAL)"=→"CAL LAB03":T15, "LAB04 (CAL)"=→"CAL LAB04":T15, "calibration file error out"=→"cal file error out":errorcluster, "LAB05 (CAL)"=→"CAL LAB05":T15)  [unwired: 9 in]
          n29 = local write "TEMP REF cal"(w24) -> ()
        }
        frame #4 {
          # "get last saved test settings from file"
          n30 = local read "Network Directory"() -> (w53:path)
          n31 = local read "C drive data root dir"() -> (w51:path)
          n32 = local read "SET LAB05-2"() -> (w83:T5)
          n33 = local read "SAMPLES"() -> (w49:dbl)
          n34 = local read "SET LAB05-1"() -> (w84:T5)
          n35 = local read "RATE (Hz)"() -> (w50:dbl)
          n36 = local read "SET LAB04-2"() -> (w85:T5)
          n37 = local read "SET LAB03-2"() -> (w82:T5)
          n38 = local read "SET LAB04-1"() -> (w86:T5)
          n39 = local read "SET LAB03-1"() -> (w81:T5)
          n40 = local read "SET LAB02-2"() -> (w80:T5)
          n41 = local read "SET LAB02-1"() -> (w79:T5)
          n42 = local read "SET LAB01-2"() -> (w78:T5)
          n43 = local read "SET LAB01-1"() -> (w77:T6)
          n44 = local read "Select COM port"() -> (w46:refnum<visa-resource-name>)
          n45 = local read "Temp Delay Lps"() -> (w45:dbl)
          n46 = local read "Mail Test File To:"() -> (w35:string)
          n47 = local read "Temp Value"() -> (w44:dbl)
          n48 = local read "Temp Test Cal"() -> (w39:dbl)
          n49 = local read "Amps Fail level"() -> (w38:dbl)
          n50 = local read "Fail Loops"() -> (w41:dbl)
          n51 = local read "Mail Test Fail"() -> (w33:bool)
          n52 = Bundle("SET LAB01-1"=w77, "SET LAB01-2"=w78, "SET LAB02-1"=w79, "SET LAB02-2"=w80, "SET LAB03-1"=w81, "SET LAB03-2"=w82, "SET LAB04-1"=w86, "SET LAB04-2"=w85, "SET LAB05-1"=w84, "SET LAB05-2"=w83, "Network Directory"=w53, "C drive data root dir"=w51, "RATE (Hz)"=w50, "SAMPLES"=w49, "Select COM port"=w46, "Temp Delay Lps"=w45, "Temp Value"=w44, "Fail Loops"=w41, "Temp Test Cal"=w39, "Amps Fail level"=w38, "Mail Test File To:"=w35, "Mail Test Fail"=w33) -> (w70:T24)  [unwired: 1 in]
          n53 = String To Path(string="c:\\crabtree\\Set Up\\") -> (path=w74:path)
          n54 = Build Path(base path=w74, name or relative path="settings.bin") -> (appended path=w72:path)
          n55 = Create Folder(path (use dialog)=w74) -> (error out=w76:errorcluster)  [unwired: 2 in, 2 out]
          n56 = call <vilib>:"Clear Errors.vi"("error in (no error)"=w76) -> ()  [unwired: 5 in, 2 out]
          n57 = Open/Create/Replace File(file path (use dialog)=w72) -> (refnum out=w69:refnum<file>, error out=w71:errorcluster)  [unwired: 5 in, 1 out]
          n58 = Read from Binary File(5:w70, 8:w71, 11:w69) -> (0:w66:errorcluster, 2:w68:T24, 3:w67:refnum<file>)  [unwired: 3 in, 1 out]
          n59 = Unbundle(w68) -> ("SET LAB01-1"=w64:T6, "SET LAB01-2"=w63:T5, "SET LAB02-1"=w62:T5, "SET LAB02-2"=w61:T5, "SET LAB03-1"=w60:T5, "SET LAB03-2"=w59:T5, "SET LAB04-1"=w58:T5, "SET LAB04-2"=w57:T5, "SET LAB05-1"=w56:T5, "SET LAB05-2"=w55:T5, "Network Directory"=w54:path, "C drive data root dir"=w52:path, "RATE (Hz)"=w47:dbl, "SAMPLES"=w48:dbl, "Select COM port"=w31:refnum<visa-resource-name>, "Temp Delay Lps"=w43:dbl, "Temp Value"=w42:dbl, "Fail Loops"=w40:dbl, "Temp Test Cal"=w37:dbl, "Amps Fail level"=w36:dbl, "Mail Test File To:"=w34:string, "Mail Test Fail"=w32:bool)
          n60 = Close File(refnum=w67, error in=w66) -> (error out=w65:errorcluster)  [unwired: 1 out]
          n61 = local write "data file error"(w65) -> ()
          n62 = local write "Temp Test Cal"(w37) -> ()
          n63 = local write "Amps Fail level"(w36) -> ()
          n64 = local write "Mail Test File To:"(w34) -> ()
          n65 = local write "Mail Test Fail"(w32) -> ()
          n66 = local write "Fail Loops"(w40) -> ()
          n67 = local write "Temp Delay Lps"(w43) -> ()
          n68 = local write "C drive data root dir"(w52) -> ()
          n69 = local write "Temp Value"(w42) -> ()
          n70 = local write "Network Directory"(w54) -> ()
          n71 = local write "SAMPLES"(w48) -> ()
          n72 = local write "RATE (Hz)"(w47) -> ()
          n73 = local write "SET LAB04-2"(w57) -> ()
          n74 = local write "SET LAB05-1"(w56) -> ()
          n75 = local write "SET LAB04-1"(w58) -> ()
          n76 = local write "SET LAB05-2"(w55) -> ()
          n77 = local write "SET LAB02-1"(w62) -> ()
          n78 = local write "SET LAB02-2"(w61) -> ()
          n79 = local write "SET LAB03-1"(w60) -> ()
          n80 = local write "SET LAB03-2"(w59) -> ()
          n81 = local write "SET LAB01-1"(w64) -> ()
          n82 = local write "SET LAB01-2"(w63) -> ()
          n83 = local write "Select COM port"(w31) -> ()
          n84 = global write "Global 1.vi" "COM port"(w31) -> ()
        }
        frame #5 {
          # "Get total resets value from file"
          n85 = String To Path(string="c:\\crabtree\\Set Up\\") -> (path=w97:path)
          n86 = Build Path(base path=w97, name or relative path="USB resets.bin") -> (appended path=w90:path)
          n87 = Create Folder(path (use dialog)=w97) -> (error out=w89:errorcluster)  [unwired: 2 in, 2 out]
          n88 = call <vilib>:"Clear Errors.vi"("error in (no error)"=w89) -> ()  [unwired: 5 in, 2 out]
          n89 = Open/Create/Replace File(file path (use dialog)=w90, operation (0:open)=T18."open or create") -> (refnum out=w95:refnum<file>, error out=w94:errorcluster)  [unwired: 4 in, 1 out]
          n90 = local read "Total USB resets"() -> (w88:dbl)
          n91 = Read from Binary File(5:w88, 8:w94, 11:w95) -> (0:w92:errorcluster, 2:w87:dbl, 3:w93:refnum<file>)  [unwired: 3 in, 1 out]
          n92 = local write "Total USB resets"(w87) -> ()
          n93 = Close File(refnum=w93, error in=w92) -> (error out=w91:errorcluster)  [unwired: 1 out]
          n94 = local write "data file error"(w91) -> ()
        }
        frame #6 {
          # "Get last saved jig cycles value from file"
          n95 = String To Path(string="c:\\crabtree\\Jig Cycles\\") -> (path=w109:path)
          n96 = Build Path(base path=w109, name or relative path="jigcycles.bin") -> (appended path=w107:path)
          n97 = Create Folder(path (use dialog)=w109) -> (error out=w111:errorcluster)  [unwired: 2 in, 2 out]
          n98 = call <vilib>:"Clear Errors.vi"("error in (no error)"=w111) -> ()  [unwired: 5 in, 2 out]
          n99 = Open/Create/Replace File(file path (use dialog)=w107) -> (refnum out=w105:refnum<file>, error out=w106:errorcluster)  [unwired: 5 in, 1 out]
          n100 = Read from Binary File(5:T9 {"LAB01-1"=0.0, "LAB01-2"=0.0, "LAB02-1"=0.0, "LAB02-2"=0.0, "LAB03-1"=0.0, "LAB03-2"=0.0, "LAB04-1"=0.0, "LAB04-2"=0.0, "LAB05-1"=0.0, "LAB05-2"=0.0} ("JIG RELAY CYCLES"), 8:w106, 11:w105) -> (0:w103:errorcluster, 2:w100:T9, 3:w104:refnum<file>)  [unwired: 3 in, 1 out]
          n101 = local write "JIG RELAY CYCLES"(w100) -> ()
          n102 = Close File(refnum=w104, error in=w103) -> (error out=w102:errorcluster)  [unwired: 1 out]
          n103 = local write "data file error"(w102) -> ()
        }
        frame #7 {
          # "Get mail settings"
          n104 = local read "Auto Mail Send"() -> (w115:bool)
          n105 = local read "MAIL SETTINGS"() -> (w119:T8)
          n106 = String To Path(string="c:\\crabtree\\Set Up\\") -> (path=w127:path)
          n107 = Build Path(base path=w127, name or relative path="mail.bin") -> (appended path=w125:path)
          n108 = Create Folder(path (use dialog)=w127) -> (error out=w129:errorcluster)  [unwired: 2 in, 2 out]
          n109 = Bundle("MAIL SETTINGS"=w119, "Auto Mail Send"=w115, "") -> (w118:T25)  [unwired: 1 in]
          n110 = call <vilib>:"Clear Errors.vi"("error in (no error)"=w129) -> ()  [unwired: 5 in, 2 out]
          n111 = Open/Create/Replace File(file path (use dialog)=w125) -> (refnum out=w123:refnum<file>, error out=w124:errorcluster)  [unwired: 5 in, 1 out]
          n112 = Read from Binary File(5:w118, 8:w124, 11:w123) -> (0:w121:errorcluster, 2:w117:T25, 3:w122:refnum<file>)  [unwired: 3 in, 1 out]
          n113 = Unbundle(w117) -> ("MAIL SETTINGS"=w116:T8, "Auto Mail Send"=w114:bool, w113:string)
          n114 = local write "Auto Mail Send"(w114) -> ()
          n115 = local write "TO (string):"(w113) -> ()
          n116 = local write "MAIL SETTINGS"(w116) -> ()
          n117 = Close File(refnum=w122, error in=w121) -> (error out=w120:errorcluster)  [unwired: 1 out]
          n118 = local write "data file error"(w120) -> ()
        }
        frame #8 {
          # "Set display status if blank"
          n119 = local read "DISP LAB03-2"() -> (w159:T4)
          n120 = local read "DISP LAB03-1"() -> (w166:T4)
          n121 = local read "DISP LAB02-2"() -> (w173:T4)
          n122 = local read "DISP LAB01-2"() -> (w186:T4)
          n123 = local read "DISP LAB01-1"() -> (w195:T4)
          n124 = local read "DISP LAB02-1"() -> (w180:T4)
          n125 = Unbundle(w159) -> ("STATUS"=w161:string)  [unwired: 2 out]
          n126 = Unbundle(w166) -> ("STATUS"=w168:string)  [unwired: 2 out]
          n127 = Unbundle(w173) -> ("STATUS"=w175:string)  [unwired: 2 out]
          n128 = Unbundle(w180) -> ("STATUS"=w182:string)  [unwired: 2 out]
          n129 = Unbundle(w186) -> ("STATUS"=w189:string)  [unwired: 2 out]
          n130 = Unbundle(w195) -> ("STATUS"=w196:string)  [unwired: 2 out]
          n131 = Equal?(x="", y=w161) -> (x = y?=w163:bool)
          n132 = Equal?(x="", y=w168) -> (x = y?=w170:bool)
          n133 = Equal?(x="", y=w175) -> (x = y?=w177:bool)
          n134 = Equal?(x="", y=w182) -> (x = y?=w184:bool)
          n135 = Equal?(x="", y=w189) -> (x = y?=w191:bool)
          n136 = Equal?(x="", y=w196) -> (x = y?=w198:bool)
          n137 = Select(t="STOP", s=w163, f=w161) -> (s? t:f=w160:string)
          n138 = Select(t="STOP", s=w170, f=w168) -> (s? t:f=w167:string)
          n139 = Select(t="STOP", s=w177, f=w175) -> (s? t:f=w174:string)
          n140 = Select(t="STOP", s=w184, f=w182) -> (s? t:f=w181:string)
          n141 = Select(t="STOP", s=w191, f=w189) -> (s? t:f=w188:string)
          n142 = Select(t="STOP", s=w198, f=w196) -> (s? t:f=w194:string)
          n143 = Bundle(cluster=w159, "STATUS"=w160) -> (w158:T4)  [unwired: 2 in]
          n144 = Bundle(cluster=w166, "STATUS"=w167) -> (w165:T4)  [unwired: 2 in]
          n145 = Bundle(cluster=w173, "STATUS"=w174) -> (w172:T4)  [unwired: 2 in]
          n146 = Bundle(cluster=w180, "STATUS"=w181) -> (w179:T4)  [unwired: 2 in]
          n147 = Bundle(cluster=w186, "STATUS"=w188) -> (w187:T4)  [unwired: 2 in]
          n148 = Bundle(cluster=w195, "STATUS"=w194) -> (w193:T4)  [unwired: 2 in]
          n149 = local write "DISP LAB01-2"(w187) -> ()
          n150 = local write "DISP LAB01-1"(w193) -> ()
          n151 = local write "DISP LAB02-1"(w179) -> ()
          n152 = local write "DISP LAB03-1"(w165) -> ()
          n153 = local write "DISP LAB02-2"(w172) -> ()
          n154 = local write "DISP LAB03-2"(w158) -> ()
          n155 = local read "DISP LAB05-2"() -> (w131:T4)
          n156 = local read "DISP LAB05-1"() -> (w138:T4)
          n157 = local read "DISP LAB04-2"() -> (w140:T4)
          n158 = local read "DISP LAB04-1"() -> (w142:T4)
          n159 = Unbundle(w131) -> ("STATUS"=w133:string)  [unwired: 2 out]
          n160 = Unbundle(w138) -> ("STATUS"=w144:string)  [unwired: 2 out]
          n161 = Unbundle(w140) -> ("STATUS"=w149:string)  [unwired: 2 out]
          n162 = Unbundle(w142) -> ("STATUS"=w154:string)  [unwired: 2 out]
          n163 = Equal?(x="", y=w133) -> (x = y?=w135:bool)
          n164 = Equal?(x="", y=w144) -> (x = y?=w146:bool)
          n165 = Equal?(x="", y=w149) -> (x = y?=w151:bool)
          n166 = Equal?(x="", y=w154) -> (x = y?=w156:bool)
          n167 = Select(t="STOP", s=w135, f=w133) -> (s? t:f=w132:string)
          n168 = Select(t="STOP", s=w146, f=w144) -> (s? t:f=w143:string)
          n169 = Select(t="STOP", s=w151, f=w149) -> (s? t:f=w148:string)
          n170 = Select(t="STOP", s=w156, f=w154) -> (s? t:f=w153:string)
          n171 = Bundle(cluster=w131, "STATUS"=w132) -> (w130:T4)  [unwired: 2 in]
          n172 = Bundle(cluster=w138, "STATUS"=w143) -> (w137:T4)  [unwired: 2 in]
          n173 = Bundle(cluster=w140, "STATUS"=w148) -> (w139:T4)  [unwired: 2 in]
          n174 = Bundle(cluster=w142, "STATUS"=w153) -> (w141:T4)  [unwired: 2 in]
          n175 = local write "DISP LAB05-2"(w130) -> ()
          n176 = local write "DISP LAB05-1"(w137) -> ()
          n177 = local write "DISP LAB04-1"(w141) -> ()
          n178 = local write "DISP LAB04-2"(w139) -> ()
        }
        frame #9 {
          w203 = 0
          w200 = FALSE
          # "initialise analog error control"
          n179 = local write "Resets Done"(0) -> ()
          n180 = local write "Auto Reset"(TRUE) -> ()
          n181 = local write "Er USB#0"(w203) -> ()
          n182 = local write "Er USB#1"(w203) -> ()
          n183 = local write "Er USB#2"(w203) -> ()
          n184 = local write "Analog error"(w200) -> ()
          n185 = local write "Reset Measuring"(w200) -> ()
          n186 = local write "Error USB #0"(w200) -> ()
          n187 = local write "Reset Error"(w200) -> ()
          n188 = local write "Error USB #1"(w200) -> ()
          n189 = local write "Error USB #2"(w200) -> ()
          n190 = local write "stop"(w200) -> ()
          n191 = local write "stop all"(w200) -> ()
        }
        frame #10 {
          # "get initial temperature values"
          n192 = stacked-sequence {
            frame #0 {
              w212 = T13 {"T1 Live"=20.0, "T1 Neut"=20.0, "T2 Live"=20.0, "T2 Neut"=20.0, "ID"=6.0, "ER"=10.0} ("LAB01 TEMP")
              n193 = local read "Select COM port"() -> (w207:refnum<visa-resource-name>)
              n194 = local write "LAB deg C"(w212) -> ()
              n195 = global write "Global display 4.vi" "LAB deg C"(w212) -> ()
              n196 = local write "OFF amps"(1.5) -> ()
              n197 = local write "ON amps"(20.0) -> ()
              n198 = local write "VOLTS"(250.0) -> ()
              n199 = local write "PF"(0.5) -> ()
